vi "RIO_I2C_PmodGYRORead.vi"(8 "error in (no error)":errorcluster, 9 "Resolution (dps)":enum16{"2000", "500", "250"}(ring), 10 "Address":enum8{"0x68", "0x69"}(ring)=enum."0x69") -> (0 "error out":errorcluster, 2 "Gyro XYZ (degrees/sec)":cluster{"X":i16, "Y":i16, "Z":i16})   [LabVIEW 2018]
doc: "Point the I2C to the 0x28 register with a 1 in the MSb slot to configure the device to read more than one byte at a time, thus 0xA8 is used.\n\nRead 6 bytes from register 0x28 and the subsequent registers. Combine the x, y, and z bytes and convert to a 2's complement signed 16 bit integer. Multiply by the corresponding resolution to get the correct gyro reading.\n\nThis VI outputs the Gyro x, y, and z values in degrees per second."
uses:
  <vilib>/MakerHub/Toolbox/LMH-Toolbox.lvlib
panel:
  in  "refnum name":string="My I2C RefNum"
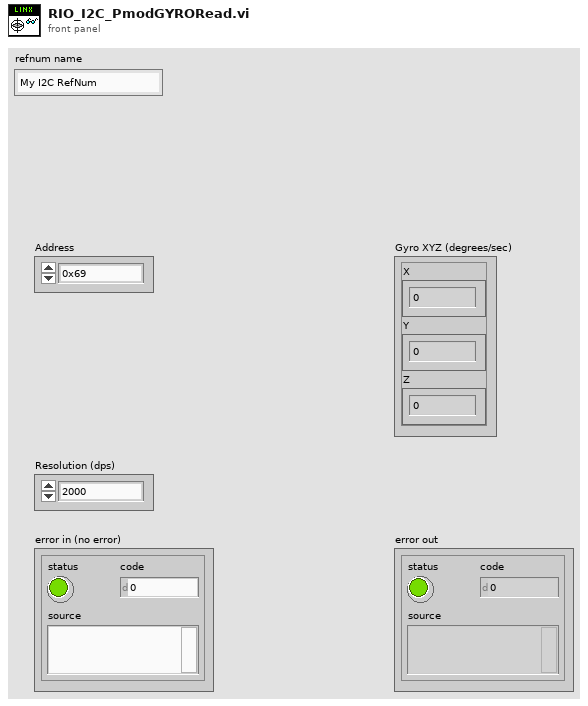
[diagram p1: front panel]
types:
  T1 = typedef "WPI_I2CDevRef.ctl" = cluster{"DevStatus":errorcluster, "Device Address":u8, "Handle":i32, "I2C Bus":T2}
  T2 = typedef "i2c_bus.ctl" = enum16{"I2C On-Board", "I2C MXP", "Invalid"}
  T3 = cluster{"Decimal I16":i16, "Decimal I16":i16, "Decimal I16":i16}
  T4 = cluster{"Decimal I16":dbl, "Decimal I16":dbl, "Decimal I16":dbl}
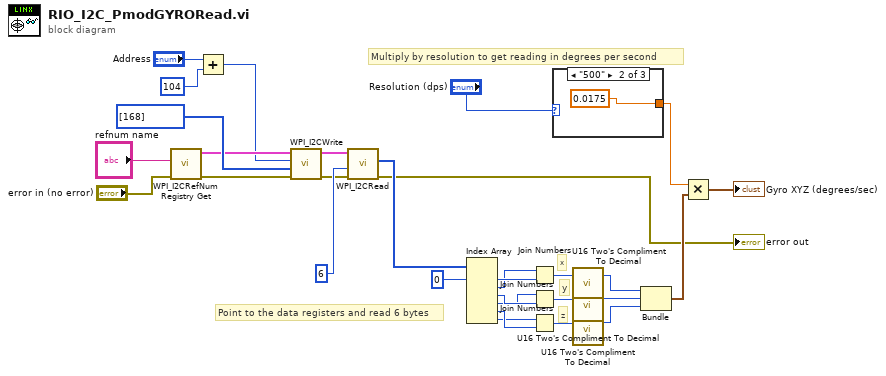
[diagram p0: block diagram]
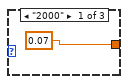
[diagram p2: hidden frame]
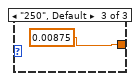
[diagram p3: hidden frame]
diagram:
  # "Multiply by resolution to get reading in degrees per second"
  # "Point to the data registers and read 6 bytes"
  # "z"
  # "y"
  # "x"
  n1 = call <vilib>:"WPI_I2CRefNum Registry Get.vi"("error in (no error)"="error in (no error)", "refnum name"="refnum name") -> ("error out"=w2:errorcluster, "I2CDevRef"=w8:T1)  [unwired: 8 in]
  n2 = Add(x="Address", y=u8 104) -> (x+y=w6:u8)
  n3 = call <vilib>:"WPI_I2CWrite.vi"("error in (no error)"=w2, "I2CDataToSend"=u8[] [168] ("Data"), "I2CRegister"=w6, "I2CDevRef"=w8) -> ("error out"=w5:errorcluster, "I2CDevRef"=w7:T1)  [unwired: 6 in]
  n4 = call <vilib>:"WPI_I2CRead.vi"("error in (no error)"=w5, "I2CBytesToRead"=u8 6 ("Bytes To Read"), "I2CDevRef"=w7) -> ("error out"=→"error out":errorcluster, "Data Out"=w11:u8[])  [unwired: 6 in, 1 out]
  n5 = Index Array(array=w11, index #1=0 ("index")) -> (element #1=w17:u8, element #2=w16:u8, element #3=w15:u8, element #4=w14:u8, element #5=w13:u8, element #6=w12:u8)  [unwired: 5 in]
  n6 = Join Numbers(hi=w16, lo=w17) -> ((hi.lo)=w22:u16)
  n7 = Join Numbers(hi=w14, lo=w15) -> ((hi.lo)=w24:u16)
  n8 = Join Numbers(hi=w12, lo=w13) -> ((hi.lo)=w23:u16)
  n9 = case shown="\"500\"" "Resolution (dps)" {
    tunnel: [0.07 0.0175 0.00875] -> w29
    frame "2000" {
    }
    frame "500" {
    }
    frame "250", Default {
    }
  }
  n10 = call <vilib>:"U16 Two's Compliment To Decimal.vi"("Two's Compliment U16"=w22) -> ("Decimal I16"=w25:i16)  [unwired: 2 in]
  n11 = call <vilib>:"U16 Two's Compliment To Decimal.vi"("Two's Compliment U16"=w24) -> ("Decimal I16"=w26:i16)  [unwired: 2 in]
  n12 = call <vilib>:"U16 Two's Compliment To Decimal.vi"("Two's Compliment U16"=w23) -> ("Decimal I16"=w27:i16)  [unwired: 2 in]
  n13 = Bundle("Decimal I16"=w25, "Decimal I16"=w26, "Decimal I16"=w27) -> (w28:T3)  [unwired: 1 in]
  n14 = Multiply(x=w29, y=w28) -> (x*y=→"Gyro XYZ (degrees/sec)":T4)
